vi "Process.vi"(8 "error in (no error)":errorcluster, 10 "pound in":refnum<class "Pound.lvclass">, 11 "qbus in":refnum<class "Qbus.lvclass">) -> (0 "error out":errorcluster)   [LabVIEW 2017, in "TimerProcess.lvlib"]
doc: "Implements timer tasks that other processes register by sending Qbus messages to those processes."
uses:
  <vilib>/addons/TimerProcess/TimerProcess.lvlib
  <vilib>/addons/Qbus/Qbus.lvclass
  <vilib>/NI/Software Watchdog/Pound/Pound.lvclass
  <vilib>/addons/TimerProcess/controls/internalTask.ctl
  <vilib>/addons/TimerProcess/controls/taskType.ctl
  <vilib>/NI/Software Watchdog/Watchdog/Watchdog.lvclass
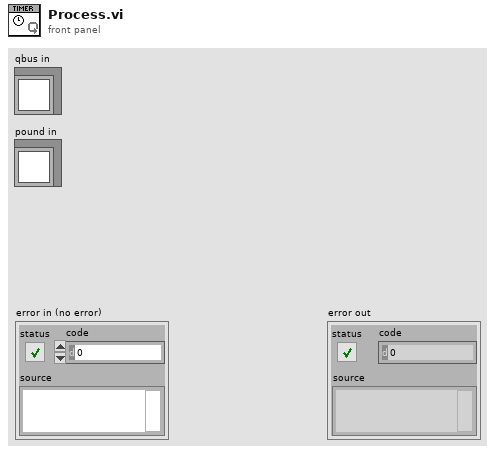
[diagram p1: front panel]
types:
  T1 = typedef "TimerProcess.lvlib/internalTask.ctl" = cluster{"Name":string, "Qbus":refnum<class "Qbus.lvclass">, "ProcessName":string, "CallBackAction":string, "CallBackValue":variant, "interval (ms)":i32, "type":T2, "state":cluster{"tickCount":u32}}
  T2 = typedef "TimerProcess.lvlib/taskType.ctl" = enum16{"single", "repeat"}
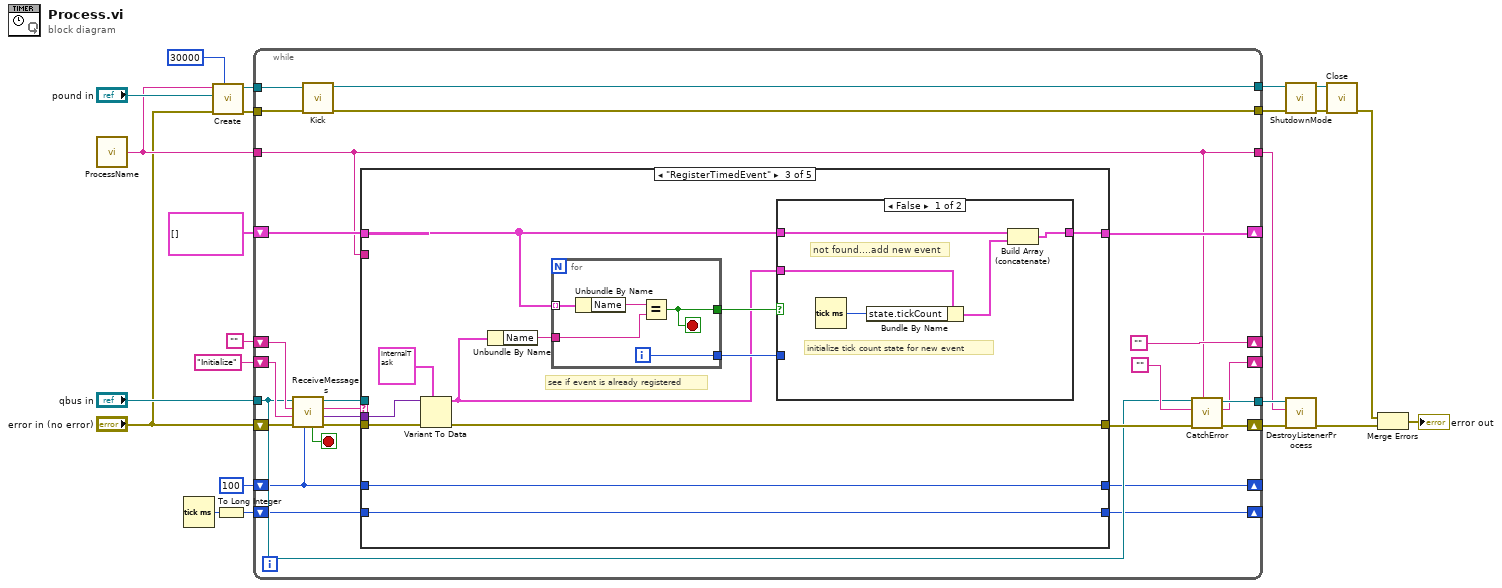
[diagram p0: block diagram]
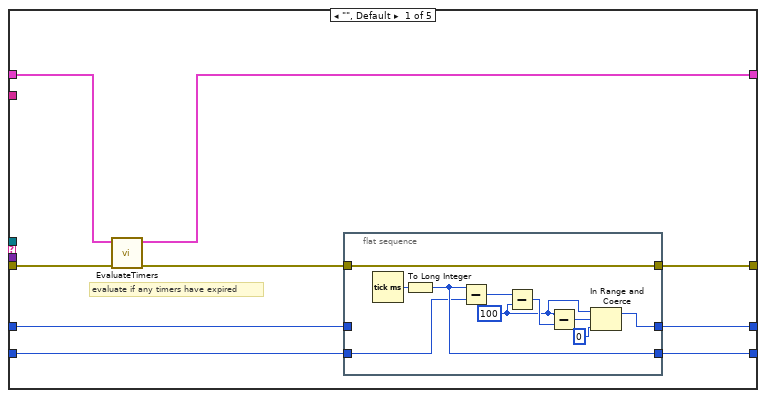
[diagram p2: hidden frame]
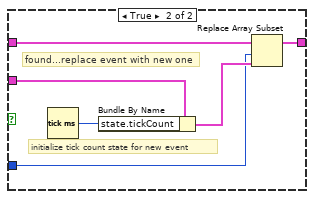
[diagram p4: hidden frame]
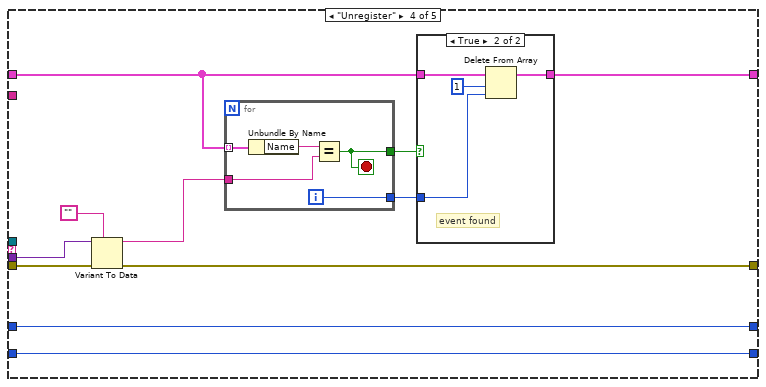
[diagram p5: hidden frame]
diagram:
  n1 = call <vilib>:"ProcessName.vi"() -> ("process name"=w13:string)  [unwired: 5 in]
  n2 = Tick Count (ms)() -> (millisecond timer value=w4:u32)
  n3 = call <vilib>:"Create.vi"("Execution Timeout (ms)"=u32 30000, "error in (no error)"="error in (no error)", "Pound"="pound in", "Name"=w13) -> ("error out"=w15:errorcluster, "Watchdog"=w14:refnum<data-value>)  [unwired: 6 in]
  n4 = To Long Integer(number=w4) -> (32bit integer=w2:i32)
  n5 = while {
    shift-right: [w44] -> _
    shift-left: T1[] [] -> [w47]
    shift-right: [""] -> _
    shift-left: "" -> [w46]
    tunnel: "qbus in" -> [w33]
    tunnel: w13 -> [w35]
    tunnel: [w38] -> w21
    tunnel: [w35] -> w20
    shift-right: [w36] -> _
    shift-left: "Initialize" -> [w40]
    tunnel: w15 -> [w32]
    tunnel: w14 -> [w31]
    tunnel: [w30] -> w8
    tunnel: [w29] -> w9
    shift-right: [w24] -> _
    shift-left: 100 ("32bit integer") -> [w25]
    shift-right: [w26] -> _
    shift-left: w2 -> [w27]
    shift-right: [w39] -> w22
    shift-left: "error in (no error)" -> [w49]
    stop <- w48 stop-if-true
    n6 = call <vilib>:"ReceiveMessages.vi"("timeout(100)"=w25, "error in (no error)"=w49, "priority action"=w40, "default action"=w46, "qbus in"=w33) -> ("error out"=w45:errorcluster, "message value"=w41:variant, "action"=w28:string, "qbus out"=w42:refnum<class "Qbus.lvclass">, "exit"=w48:bool)  [unwired: 2 in]
    n7 = call <vilib>:"Kick.vi"("error in (no error)"=w32, "Watchdog"=w31) -> ("error out"=w29:errorcluster, "Watchdog"=w30:refnum<data-value>)  [unwired: 8 in]
    n8 = case shown="\"RegisterTimedEvent\"" w28 {
      tunnel: w47 -> [w57 w72 w78 w105 w125]
      tunnel: w45 -> [w58 w69 w84 w110 w122]
      tunnel: w42 -> [_ _ _ _ _]
      tunnel: [w54 w69 w76 w103 w122] -> w34
      tunnel: [w56 w72 w75 w104 w125] -> w44
      tunnel: w41 -> [_ _ w82 w109 _]
      tunnel: w35 -> [_ _ _ _ _]
      tunnel: w25 -> [w53 w71 w74 w102 w124]
      tunnel: w27 -> [w52 w70 w73 w101 w123]
      tunnel: [w51 w70 w73 w101 w123] -> w26
      tunnel: [w50 w71 w74 w102 w124] -> w24
      frame "", Default {
        # "evaluate if any timers have expired"
        n9 = call <vilib>:"EvaluateTimers.vi"("error in (no error)"=w58, "timer in"=w57) -> ("error out"=w55:errorcluster, "timer out"=w56:T1[])  [unwired: 8 in]
        n10 = flat-sequence {
          tunnel: [w68] -> w54
          tunnel: w55 -> [w68]
          tunnel: w53 -> [_]
          tunnel: [w66] -> w51
          tunnel: w52 -> [w65]
          tunnel: [w59] -> w50
          frame #0 {
            w61 = 100 ("32bit integer")
            n11 = Tick Count (ms)() -> (millisecond timer value=w67:u32)
            n12 = To Long Integer(number=w67) -> (32bit integer=w66:i32)
            n13 = Subtract(x=w66, y=w65) -> (x-y=w64:i32)
            n14 = Subtract(x=w64, y=w61) -> (x-y=w63:i32)
            n15 = Subtract(x=w61, y=w63) -> (x-y=w62:i32)
            n16 = In Range and Coerce(upper limit=w61, x=w62, lower limit=0) -> (coerced(x)=w59:i32)  [unwired: 1 out]
          }
        }
      }
      frame "Initialize" {
      }
      frame "RegisterTimedEvent" {
        # "see if event is already registered"
        n17 = Variant To Data(error in=w84, type=T1 {"Name"="", "Qbus"=refnum, "ProcessName"="", "CallBackAction"="", "CallBackValue"=variant, "interval (ms)"=0, "type"=enum."single", "state"={"tickCount"=0}} ("Task"), Variant=w82) -> (data=w77:T1, error out=w76:errorcluster)
        n18 = Unbundle By Name(w77) -> ("Name"=w79:string)
        n19 = for {
          tunnel: w78 -> [w100] mode=indexing
          tunnel: w79 -> [w98]
          tunnel: [w97] -> w80
          tunnel: [w96] -> w81
          i -> [w96]
          stop <- w97 stop-if-true
          n20 = Unbundle By Name(w100) -> ("Name"=w99:string)
          n21 = Equal?(x=w99, y=w98) -> (x = y?=w97:bool)
        }
        n22 = case shown="False" w80 {
          tunnel: [w87 w92] -> w75
          tunnel: w78 -> [w86 w93]
          tunnel: w77 -> [w85 w94]
          tunnel: w81 -> [_ w90]
          frame False {
            # "not found....add new event"
            # "initialize tick count state for new event"
            n23 = Tick Count (ms)() -> (millisecond timer value=w89:u32)
            n24 = Bundle By Name(cluster=w85, "state.tickCount"=w89) -> (w88:T1)
            n25 = Build Array (concatenate)(w86, w88) -> (w87:T1[])
          }
          frame True {
            # "found...replace event with new one"
            # "initialize tick count state for new event"
            n26 = Tick Count (ms)() -> (millisecond timer value=w95:u32)
            n27 = Bundle By Name(cluster=w94, "state.tickCount"=w95) -> (w91:T1)
            n28 = Replace Array Subset(array=w93, new element=w91, index=w90) -> (w92:T1[])
          }
        }
      }
      frame "Unregister" {
        n29 = Variant To Data(error in=w110, type="", Variant=w109) -> (data=w106:string, error out=w103:errorcluster)
        n30 = for {
          tunnel: w105 -> [w121] mode=indexing
          tunnel: w106 -> [w119]
          tunnel: [w118] -> w107
          tunnel: [w117] -> w108
          i -> [w117]
          stop <- w118 stop-if-true
          n31 = Unbundle By Name(w121) -> ("Name"=w120:string)
          n32 = Equal?(x=w120, y=w119) -> (x = y?=w118:bool)
        }
        n33 = case shown="True" w107 {
          tunnel: w105 -> [w112 w116]
          tunnel: w108 -> [_ w114]
          tunnel: [w112 w115] -> w104
          frame False {
            # "event not found"
          }
          frame True {
            # "event found"
            n34 = Delete From Array(array=w116, length=1, index=w114) -> (array with subset deleted=w115:T1[])  [unwired: 1 out]
          }
        }
      }
      frame "Exit" {
      }
    }
    n35 = call <vilib>:"CatchError.vi"("source"=w35, "error in (no error)"=w34, "next action in"="", "Qbus in"=w33) -> ("error out"=w39:errorcluster, "next action out"=w36:string, "Qbus out"=w38:refnum<class "Qbus.lvclass">)  [unwired: 5 in]
  }
  n36 = call <vilib>:"ShutdownMode.vi"("error in (no error)"=w9, "Watchdog"=w8) -> ("error out"=w10:errorcluster, "Watchdog"=w11:refnum<data-value>)  [unwired: 8 in]
  n37 = call <vilib>:"DestroyListenerProcess.vi"("error in (no error)"=w22, "process name"=w20, "Qbus in"=w21) -> ("error in (no error)"=w6:errorcluster)  [unwired: 7 in, 1 out]
  n38 = call <vilib>:"Close.vi"("error in (no error)"=w10, "Watchdog"=w11) -> ("error out"=w7:errorcluster)  [unwired: 9 in]
  n39 = Merge Errors(w7, w6) -> (→"error out":errorcluster)
